vi "GetTemplatePath.vi"(0 "reference in":refnum<class "ClassWriterNative.lvclass">, 1 "ClassTemplateSubDirectory":string, 5 "error in (no error)":errorcluster) -> (14 "reference out":refnum<class "ClassWriterNative.lvclass">, 15 "FolderPathOut":path, 17 "MethodTemplatePathOut":path, 18 "TemplateSettings":T1, 19 "error out":errorcluster)   [LabVIEW 2020, in "ClassWriterNative.lvclass"]
uses:
  <resource>/Framework/Providers/Open_GDS/ClassProviders/Provider_LvNativeClass/ClassWriterNative_class/ClassWriterNative.lvclass
  <resource>/Framework/Providers/Open_GDS/ClassProviders/Provider_BaseClassInterface/ClassWriter_class/TemplateSettings.ctl
  <resource>/Framework/Providers/Open_GDS/ClassProviders/Provider_BaseClassInterface/ClassWriter_class/ClassWriter.lvclass
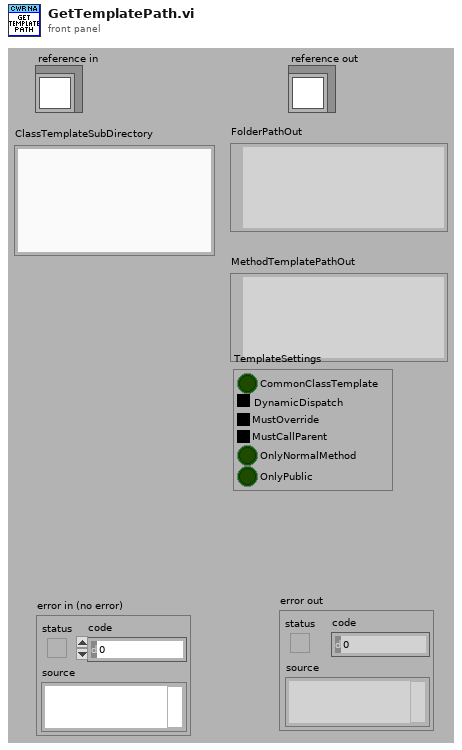
[diagram p1: front panel]
types:
  T1 = typedef "ClassWriter.lvclass/TemplateSettings.ctl" = cluster{"CommonClassTemplate":bool, "DynamicDispatch":enum8{"False", "True", "Mixed"}, "MustOverride":enum8{"False", "True", "Mixed"}, "MustCallParent":enum8{"False", "True", "Mixed"}, "OnlyNormalMethod":bool, "OnlyPublic":bool}
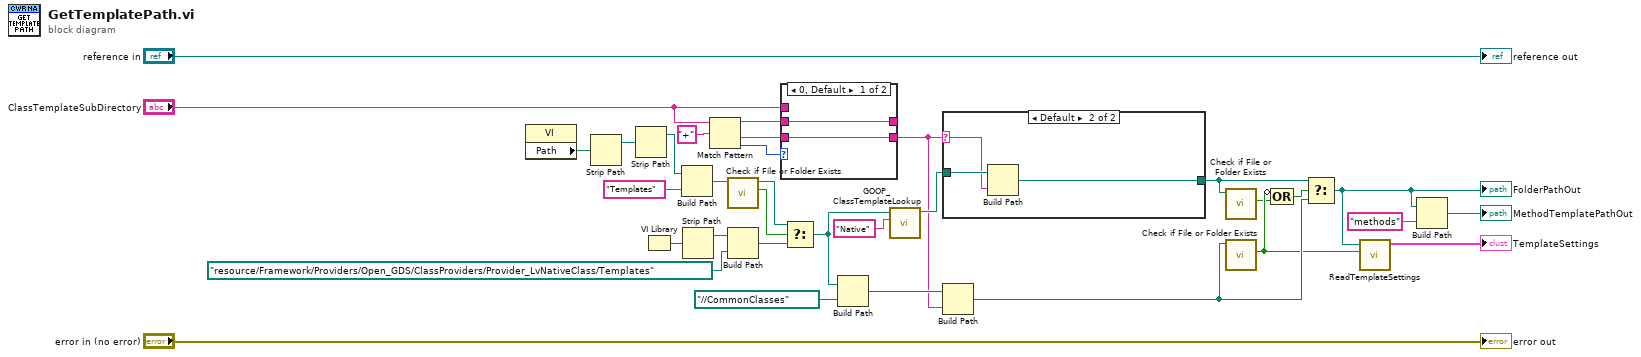
[diagram p0: block diagram]
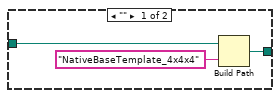
[diagram p3: hidden frame]
diagram:
  n1 = property class="VI"() -> ("Path"=w31:path)  [unwired: 2 in, 2 out]
  n2 = Strip Path(path=w31) -> (stripped path=w29:path)  [unwired: 1 out]
  n3 = Strip Path(path=w29) -> (stripped path=w33:path)  [unwired: 1 out]
  n4 = VI Library() -> (path=w25:path)
  n5 = Build Path(base path=w33, name or relative path="Templates") -> (appended path=w26:path)
  n6 = Strip Path(path=w25) -> (stripped path=w20:path)  [unwired: 1 out]
  n7 = Match Pattern(string="ClassTemplateSubDirectory", regular expression="+") -> (before substring=w16:string, after substring=w19:string, offset past match=w18:i32)  [unwired: 1 in, 1 out]
  n8 = call <vilib>:"Check if File or Folder Exists.vi"("path"=w26) -> ("file or folder exists?"=w28:bool, "dup path"=w27:path)  [unwired: 8 in, 1 out]
  n9 = Build Path(base path=w20, name or relative path=path "resource/Framework/Providers/Open_GDS/ClassProviders/Provider_LvNativeClass/Templates") -> (appended path=w24:path)
  n10 = case shown="0, Default" w18 {
    tunnel: "ClassTemplateSubDirectory" -> [_ w36]
    tunnel: [w35 w36] -> w9
    tunnel: w19 -> [w35 _]
    tunnel: [w34 _] -> _
    tunnel: w16 -> [w34 _]
    frame 0, Default {
    }
    frame -1 {
    }
  }
  n11 = Select(t=w27, s=w28, f=w24) -> (s? t:f=w11:path)
  n12 = Build Path(base path=w11, name or relative path=path "../../CommonClasses") -> (appended path=w10:path)
  n13 = call <resource>:"GOOP_ClassTemplateLookup.vi"("ClassType"="Native", "ClassTemplateFolderIn"=w11) -> ("ClassTemplateFolderOut"=w14:path)  [unwired: 9 in]
  n14 = case shown="Default" w9 {
    selector: w9 -> [_ w40]
    tunnel: w14 -> [w39 w42]
    tunnel: [w38 w41] -> w12
    frame "" {
      n15 = Build Path(base path=w39, name or relative path="NativeBaseTemplate_4x4x4") -> (appended path=w38:path)
    }
    frame Default {
      n16 = Build Path(base path=w42, name or relative path=w40) -> (appended path=w41:path)
    }
  }
  n17 = Build Path(base path=w10, name or relative path=w9) -> (appended path=w4:path)
  n18 = call <vilib>:"Check if File or Folder Exists.vi"("path"=w12) -> ("file or folder exists?"=w2:bool)  [unwired: 8 in, 2 out]
  n19 = call <vilib>:"Check if File or Folder Exists.vi"("path"=w4) -> ("file or folder exists?"=w3:bool)  [unwired: 8 in, 2 out]
  n20 = Compound Arithmetic op=OR(invert w3, w2) -> (w1:bool)
  n21 = Select(t=w12, s=w1, f=w4) -> (s? t:f=w5:path)
  "FolderPathOut" <- w5
  n22 = call <resource>:"ReadTemplateSettings.vi"("CommonClassTemplate"=w3, "TemplateFolder"=w5) -> ("TemplateSettings"=→"TemplateSettings":T1)  [unwired: 9 in]
  n23 = Build Path(base path=w5, name or relative path="methods") -> (appended path=→"MethodTemplatePathOut":path)
  "error out" <- "error in (no error)"
  "reference out" <- "reference in"
